vi "Driver Globals--FGV.vi"(7 "?":T4=enum."Get Variable References", 8 "error in":errorcluster, 9 "Name":string, 11 "Driver Settings In":T1={"Waveform Length"=0, "Data Size"=enum."16 Bit (Signed Short)", "DTACQ Connection Data"={"Description"="", "Address"="", "Port"=0, "timeout (ms)"=5000, "Termination Character"="\n", "TCP Connection Reference"=refnum, "Open Connection"=FALSE}}) -> (0 "error out":errorcluster, 1 "Searched Reference":refnum<k21>, 2 "Variable References":refnum<k21>[](array[refnum]), 3 "Driver Settings Out":T1={"Waveform Length"=0, "Data Size"=enum."16 Bit (Signed Short)", "DTACQ Connection Data"={"Description"="", "Address"="", "Port"=0, "timeout (ms)"=5000, "Termination Character"="\n", "TCP Connection Reference"=refnum, "Open Connection"=FALSE}})   [LabVIEW 2017, in "DTACQ - Network Enabled Device Driver.lvlib"]
uses:
  DTACQ - Network Enabled Device Driver.lvlib
  FGV Operaions--Enum.ctl
  Driver Global Settings--Typedef.ctl
  Communications/Typedefs/Data Size--Enum.ctl
  Communications/Typedefs/DTACQ Connection Data--Cluster.ctl
  Network Shared Variables/Typedefs/X and Y Variant Arrays--Cluster.ctl
  Network Shared Variables/Shared Variables Library.lvlib
  <resource>/objmgr/ni.var.rc
  Communications/Communications Library.lvlib
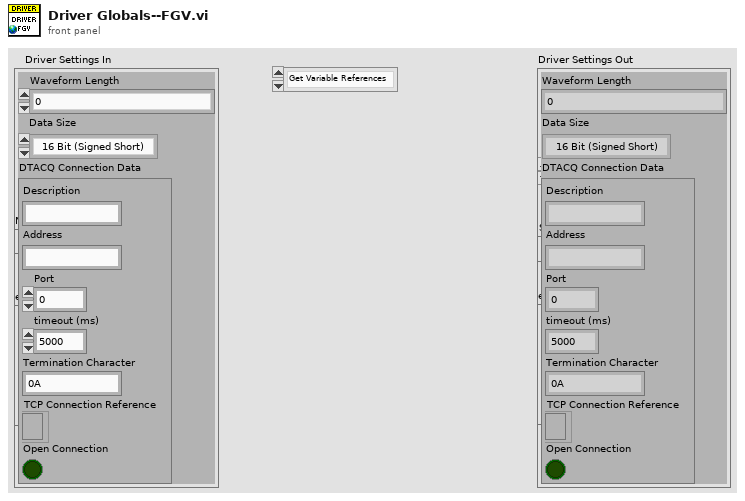
[diagram p1: front panel]
types:
  T1 = typedef "DTACQ - Network Enabled Device Driver.lvlib/Driver Global Settings--Typedef.ctl" = cluster{"Waveform Length":i32, "Data Size":T2, "DTACQ Connection Data":T3}
  T2 = typedef "Communications Library.lvlib/Data Size--Enum.ctl" = enum16{"16 Bit (Signed Short)", "32 Bit (Signed Long)"}
  T3 = typedef "Communications Library.lvlib/DTACQ Connection Data--Cluster.ctl" = cluster{"Description":string, "Address":string, "Port":u16, "timeout (ms)":i32, "Termination Character":string, "TCP Connection Reference":refnum<k5>, "Open Connection":bool}
  T4 = typedef "DTACQ - Network Enabled Device Driver.lvlib/FGV Operaions--Enum.ctl" = enum16{"Get Driver Settings", "Set Driver Settings", "Search Variable Names", "Close Connections", "Open Connections", "Get Variable References", "Set Variable References", "Clear"}
  T5 = typedef "Shared Variables Library.lvlib/X and Y Variant Arrays--Cluster.ctl" = cluster{"X-Data":variant[], "Y-Data":variant[]}
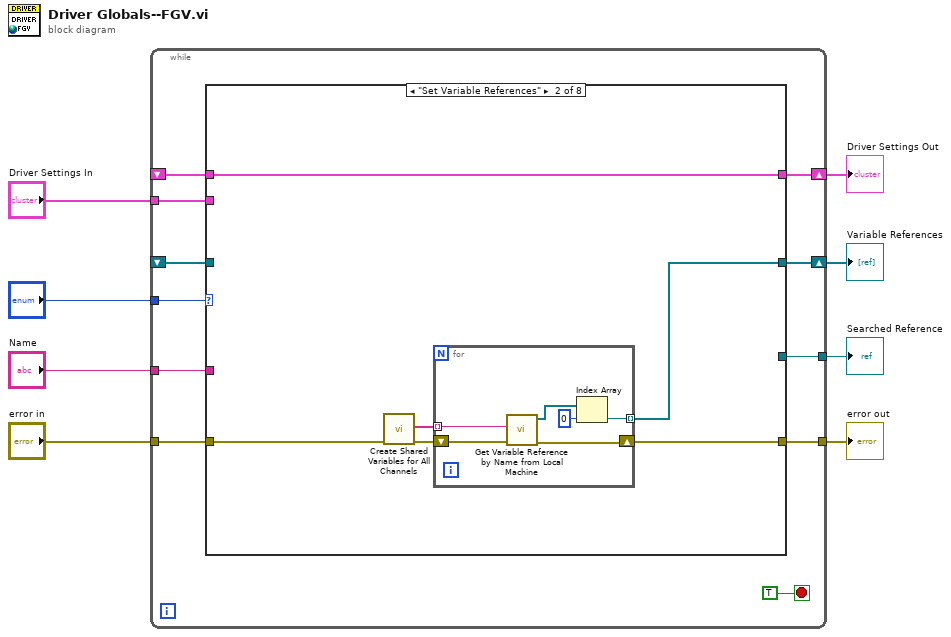
[diagram p0: block diagram]
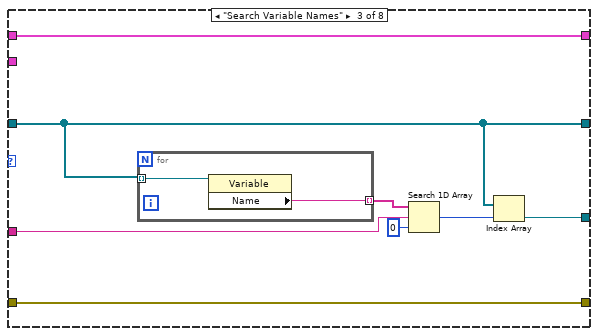
[diagram p3: hidden frame]
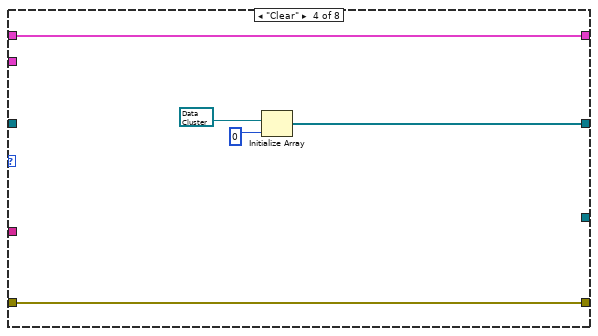
[diagram p4: hidden frame]
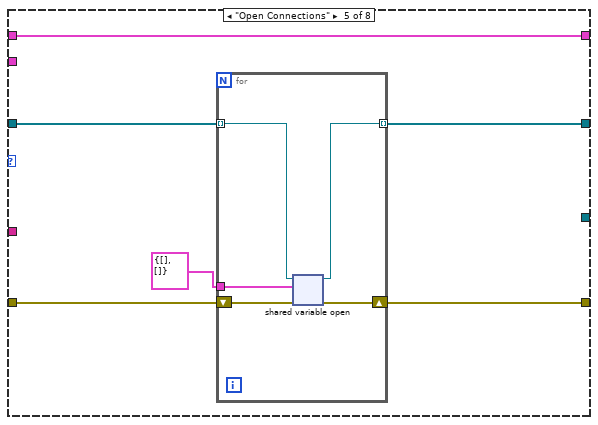
[diagram p5: hidden frame]
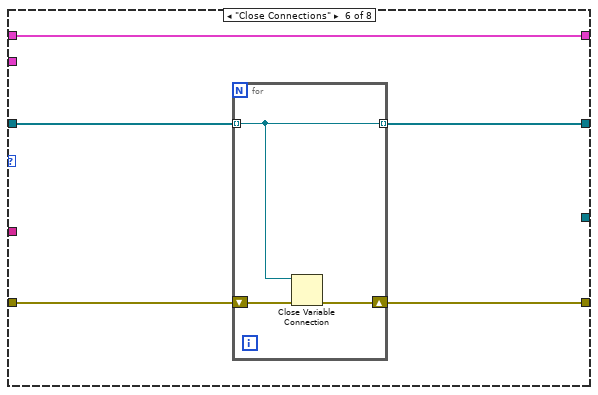
[diagram p6: hidden frame]
diagram:
  n1 = while {
    tunnel: "?" -> [w18]
    shift-right: [w17] -> w6
    shift-left: _ -> [w16]
    tunnel: [w15] -> w3
    tunnel: "error in" -> [w14]
    tunnel: "Name" -> [w13]
    tunnel: [w12] -> w4
    shift-right: [w11] -> w2
    shift-left: _ -> [w10]
    tunnel: "Driver Settings In" -> [w9]
    stop <- TRUE stop-if-true
    n2 = case shown="\"Set Variable References\"" w18 {
      tunnel: [w22 w26 w39 w48 w52 w62 w70 w72] -> w17
      tunnel: w16 -> [w22 _ w39 _ w53 w63 w70 w72]
      tunnel: [w21 w25 w36 w46 w54 w64 w71 w74] -> w15
      tunnel: w14 -> [w21 w24 w36 w46 w55 w65 w71 w74]
      tunnel: w13 -> [_ _ w41 _ _ _ _ _]
      tunnel: [_ _ w37 _ _ _ _ _] -> w12
      tunnel: [w20 w23 w35 w45 w50 w61 w69 w73] -> w11
      tunnel: w10 -> [w20 w23 w35 w45 w50 w61 _ w73]
      tunnel: w9 -> [_ _ _ _ _ _ w69 _]
      frame "Get Variable References", Default {
      }
      frame "Set Variable References" {
        n3 = call "Create Shared Variables for All Channels.vi"("error in"=w24) -> ("error out"=w28:errorcluster, "Variable Names"=w27:string[])  [unwired: 9 in]
        n4 = for {
          shift-right: [w33] -> w25
          shift-left: w28 -> [w34]
          tunnel: w27 -> [w32] mode=indexing
          tunnel: [w29] -> w26 mode=indexing
          n5 = call "Get Variable Reference by Name from Local Machine.vi"("error in"=w34, "Search"=w32) -> ("error out"=w33:errorcluster, "Variable References Out"=w31:refnum<k21>[])  [unwired: 7 in, 1 out]
          n6 = Index Array(array=w31, index=0) -> (element=w29:refnum<k21>)
        }
      }
      frame "Search Variable Names" {
        n7 = for {
          tunnel: w39 -> [w44] mode=indexing
          tunnel: [w43] -> w42 mode=indexing
          n8 = property class="Variable"(reference=w44) -> ("Name"=w43:string)  [unwired: 1 in, 2 out]
        }
        n9 = Search 1D Array(1D array=w42, element=w41, start index (0)=0) -> (index of element=w38:i32)
        n10 = Index Array(array=w39, index=w38) -> (element=w37:refnum<k21>)
      }
      frame "Clear" {
        n11 = Initialize Array(refnum<k21> refnum, 0 ("dimension size")) -> (w48:refnum<k21>[])
      }
      frame "Open Connections" {
        n12 = for {
          shift-right: [w56] -> w54
          shift-left: w55 -> [w60]
          tunnel: w53 -> [w59] mode=indexing
          tunnel: [w58] -> w52 mode=indexing
          tunnel: T5 {"X-Data"=[], "Y-Data"=[]} ("Data Cluster") -> [w57]
          n13 = shared-variable-open(w59, w60, w57) -> (w58:refnum<k21>, w56:errorcluster)
        }
      }
      frame "Close Connections" {
        n14 = for {
          shift-right: [w67] -> w64
          shift-left: w65 -> [w68]
          tunnel: w63 -> [w66] mode=indexing
          tunnel: [w66] -> w62 mode=indexing
          n15 = Close Variable Connection(8:w68, 11:w66) -> (0:w67:errorcluster)
        }
      }
      frame "Set Driver Settings" {
      }
      frame "Get Driver Settings" {
      }
    }
  }
  "Variable References" <- w6
  "Searched Reference" <- w4
  "error out" <- w3
  "Driver Settings Out" <- w2
